vi "BotSpeak_AskDevice.vi"(3 "Bot Settings":T2={"Address"="", "Reply EOF"="", "Hardware"="", "Retries"=3, "Timeout"=10, "Open?"=FALSE}) -> (1 "Bot Settings out":T2)   [LabVIEW 2012]
uses:
  <userlib>/botspeak/VIs/Direct/BotSpeak_Control.ctl
  <vilib>/Platform/browser.llb/Open URL in Default Browser (string).vi
  <userlib>/botspeak/VIs/SubVIs/BotSpeak_Globals.vi
panel:
  out "Finished":bool
  in  "View":enum32{"Normal", "Testing"}(tab)
  out "Help":string
  in  "Hardware":u16(ring) items=["Arduino Uno", "BeagleBone Serial", "BeagleBone", "Console Only", "EV3", "EvalRIO", "Galileo", "Launchpad", "MyRIO", "PICAXE 80M", "Raspberry Pi", "Thymio"]
  in  "Done":bool
  in  "Cancel":bool
  in  "Connection":T1(tab)
  in  "IP Address":string(combo)
  in  "VISA":u16(ring)
  in  "Test":bool
  in  "Goto URL":bool
  out "URL":string
  out "Status":string
  out "firmware":string
  in  "Back":bool
  out "List":string[](array[string])
  # "For More Help:"
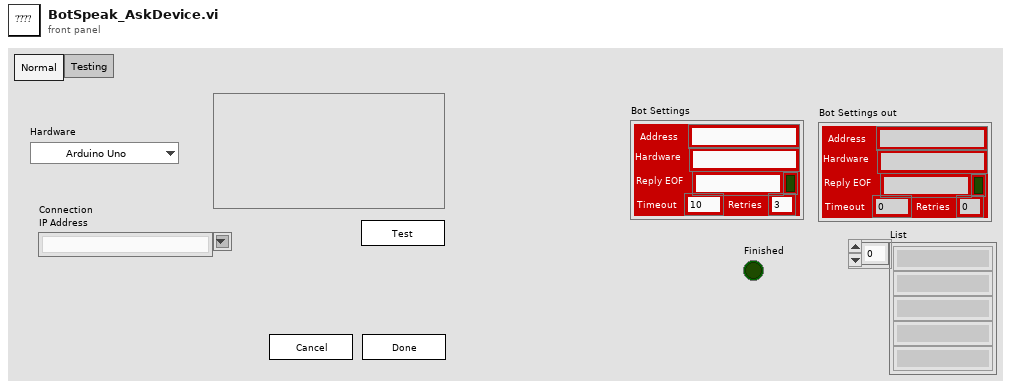
[diagram p1: front panel]
types:
  T1 = enum32{"TCPIP", "Serial", "Undefined", "Console"}
  T2 = typedef "BotSpeak_Control.ctl" = cluster{"Address":string, "Reply EOF":string, "Hardware":string, "Retries":i8, "Timeout":i32, "Open?":bool}
  T3 = typedef "BotSpeak.HardwareSpecs.ctl" = cluster{"Hardware Name":string, "Hardware URL":string, "ComType":enum16{"Undefined", "HTTP", "Serial", "TCPIP", "Console"}, "TCP Port":i32, "DefaultAddress":string, "Retries":i32, "Translate":enum16{"None", "Tiny", "URAPI"}, "MaxScriptSize":i32, "MaxVarNumber":i32, "StartupWait":i32, "Patience":i32, "Startup Patience":i32, "Hardware Help":string, "Com Protocol":string, "Translator":cluster{"BotSpeak CMD":string, "CMD out":string}[], "Init Code":string, "Variable Format":enum16{"INT", "FLOAT", "FIXED"}, "username":string, "password":string}
  T4 = enum16{"Undefined", "HTTP", "Serial", "TCPIP", "Console"}
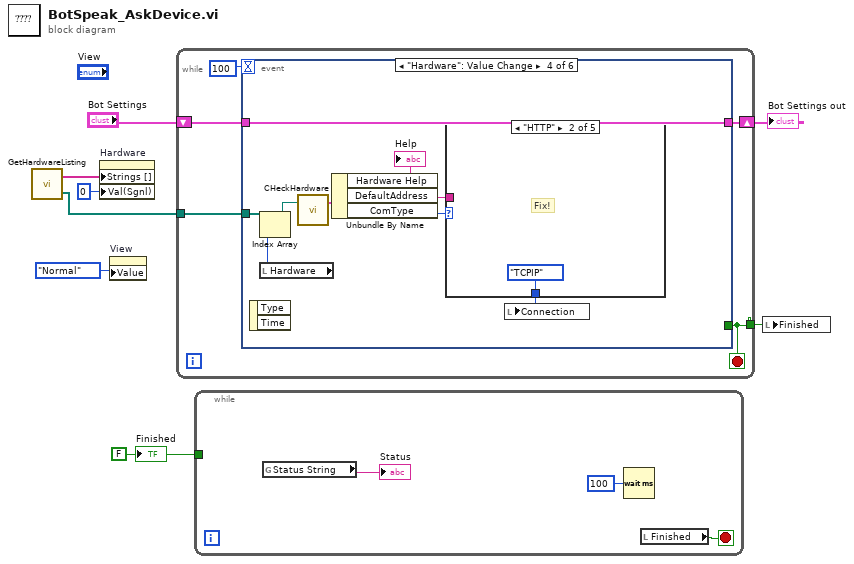
[diagram p0: block diagram]
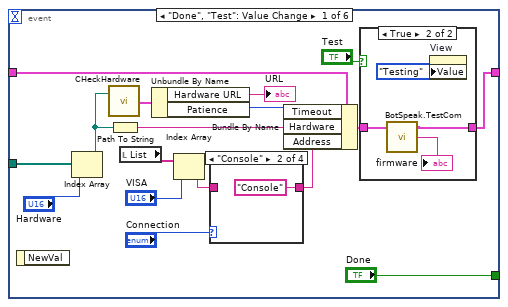
[diagram p2: hidden frame]
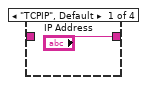
[diagram p3: hidden frame]
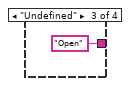
[diagram p4: hidden frame]
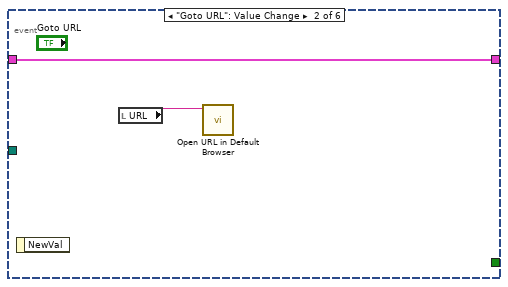
[diagram p7: hidden frame]
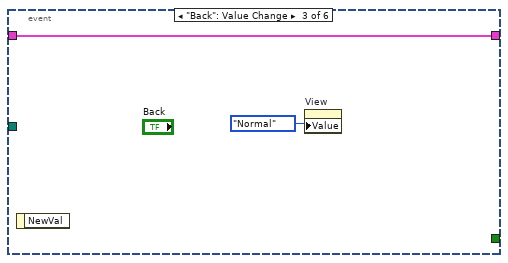
[diagram p8: hidden frame]
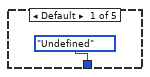
[diagram p9: hidden frame]
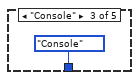
[diagram p10: hidden frame]
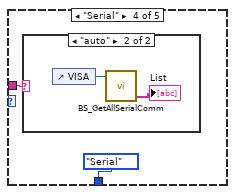
[diagram p11: hidden frame]
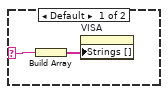
[diagram p12: hidden frame]
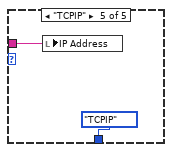
[diagram p13: hidden frame]
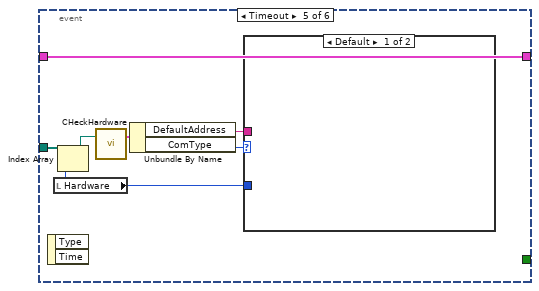
[diagram p14: hidden frame]
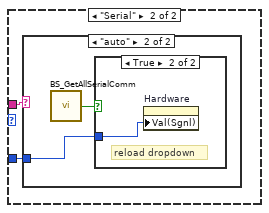
[diagram p15: hidden frame]
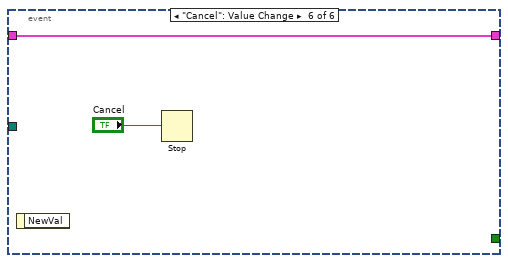
[diagram p18: hidden frame]
diagram:
  w3 = FALSE ("Finished")
  n1 = call <userlib>:"GetHardwareListing.vi"() -> ("Devices"=w1:path[], "Array"=w2:string[])  [unwired: 2 in]
  n2 = property on="Hardware" class="Ring (strict)"("Strings []"=w2, "Val(Sgnl)"=u16 0 ("Value (Signaling)")) -> ()  [unwired: 2 in, 2 out]
  n3 = property on="View" class="TabCtl (strict)"("Value"=enum32{"Normal", "Testing"}."Normal" ("View")) -> ()  [unwired: 2 in, 2 out]
  n4 = while {
    tunnel: w1 -> [w12]
    tunnel: [w9] -> w4
    shift-right: [w13] -> w8
    shift-left: "Bot Settings" -> [w11]
    stop <- w9 stop-if-true
    n5 = event shown="[3] \"Hardware\": Value Change" {
      selector: _ -> [_ _ _ _ _ _]
      dyn-events: _ -> [_ _ _ _ _ _]
      timeout: 100 -> [_ _ _ _ _ _]
      tunnel: w12 -> [w30 _ _ w52 w70 _]
      tunnel: w11 -> [w28 w40 w42 w44 w64 w76]
      tunnel: [w20 w40 w42 w44 w64 w76] -> w13
      tunnel: ["Done" _ _ _ _ _] -> w9
      event "Done", "Test": Value Change {
        n6 = event-data() -> ()  [unwired: 1 in, 1 out]
        n7 = Index Array(array=w30, index="Hardware") -> (element=w19:path)
        n8 = call <userlib>:"CHeckHardware.vi"("Hardware"=w19) -> ("HardwareSpecs"=w23:T3)  [unwired: 2 in]
        n9 = Path To String(path=w19) -> (string=w14:string)
        n10 = local read "List"() -> (w25:string[])
        n11 = Unbundle By Name(w23) -> ("Hardware URL"=→"URL":string, "Patience"=w15:i32)
        n12 = Index Array(array=w25, index="VISA") -> (element=w16:string)
        n13 = case shown="\"Console\"" "Connection" {
          tunnel: ["IP Address" "Console" ("Intf Inst Name") "Open" ("Intf Inst Name") w34] -> w17
          tunnel: w16 -> [_ _ _ w34]
          frame "TCPIP", Default {
          }
          frame "Console" {
          }
          frame "Undefined" {
          }
          frame "Serial" {
          }
        }
        n14 = Bundle By Name(cluster=w28, "Timeout"=w15, "Hardware"=w14, "Address"=w17) -> (w21:T2)
        n15 = case shown="True" "Test" {
          tunnel: w21 -> [w35 w38]
          tunnel: [w35 w37] -> w20
          frame False {
          }
          frame True {
            n16 = call <userlib>:"BotSpeak.TestCom.vi"("Bot Settings"=w38) -> ("Bot Settings out"=w37:T2, "firmware"=→"firmware":string)  [unwired: 1 in, 1 out]
            n17 = property on="View" class="TabCtl (strict)"("Value"=enum32{"Normal", "Testing"}."Testing" ("View")) -> ()  [unwired: 2 in, 2 out]
          }
        }
      }
      event "Goto URL": Value Change {
        n18 = event-data() -> ()  [unwired: 1 in, 1 out]
        n19 = local read "URL"() -> (w41:string)
        n20 = call-poly <vilib>:"Open URL in Default Browser.vi"("URL"=w41) -> ()  [unwired: 5 in, 2 out]
      }
      event "Back": Value Change {
        n21 = event-data() -> ()  [unwired: 1 in, 1 out]
        n22 = property on="View" class="TabCtl (strict)"("Value"=enum32{"Normal", "Testing"}."Normal" ("View")) -> ()  [unwired: 2 in, 2 out]
      }
      event "Hardware": Value Change {
        n23 = event-data() -> ()  [unwired: 1 in, 2 out]
        n24 = local read "Hardware"() -> (w46:u16)
        n25 = Index Array(array=w52, index=w46) -> (element=w51:path)
        n26 = call <userlib>:"CHeckHardware.vi"("Hardware"=w51) -> ("HardwareSpecs"=w50:T3)  [unwired: 2 in]
        n27 = Unbundle By Name(w50) -> ("Hardware Help"=→"Help":string, "DefaultAddress"=w47:string, "ComType"=w49:T4)
        n28 = case shown="\"HTTP\"" w49 {
          tunnel: [T1."Undefined" ("Connection") T1."TCPIP" ("Connection") T1."Console" ("Connection") enum32{"TCPIP", "Serial", "Undefined"}."Serial" ("Tabs") enum32{"TCPIP", "Serial", "Undefined"}."TCPIP" ("Tabs")] -> w48
          tunnel: w47 -> [_ _ _ w56 w62]
          frame Default {
          }
          frame "HTTP" {
            # "Fix!"
          }
          frame "Console" {
          }
          frame "Serial" {
            n29 = case shown="\"auto\"" w56 {
              selector: w56 -> [w59 _]
              frame Default {
                n30 = Build Array(w59) -> (w58:string[])
                n31 = property on="VISA" class="Ring (strict)"("Strings []"=w58) -> ()  [unwired: 2 in, 2 out]
              }
              frame "auto" {
                n32 = control-ref of="VISA"() -> (w61:refnum<vi>)
                n33 = call <userlib>:"BS_GetAllSerialComm.vi"("reference"=w61) -> ("List"=→"List":string[])  [unwired: 1 in, 2 out]
              }
            }
          }
          frame "TCPIP" {
            n34 = local write "IP Address"(w62) -> ()
          }
        }
        n35 = local write "Connection"(w48) -> ()
      }
      event Timeout {
        n36 = event-data() -> ()  [unwired: 1 in, 2 out]
        n37 = local read "Hardware"() -> (w65:u16)
        n38 = Index Array(array=w70, index=w65) -> (element=w69:path)
        n39 = call <userlib>:"CHeckHardware.vi"("Hardware"=w69) -> ("HardwareSpecs"=w68:T3)  [unwired: 2 in]
        n40 = Unbundle By Name(w68) -> ("DefaultAddress"=w66:string, "ComType"=w67:T4)
        n41 = case shown="Default" w67 {
          tunnel: w66 -> [_ w72]
          tunnel: w65 -> [_ w71]
          frame Default {
          }
          frame "Serial" {
            n42 = case shown="\"auto\"" w72 {
              tunnel: w71 -> [_ w73]
              frame Default {
              }
              frame "auto" {
                n43 = call <userlib>:"BS_GetAllSerialComm.vi"() -> ("new?"=w74:bool)  [unwired: 2 in, 2 out]
                n44 = case shown="True" w74 {
                  tunnel: w73 -> [_ w75]
                  frame False {
                  }
                  frame True {
                    # "reload dropdown"
                    n45 = property on="Hardware" class="Ring (strict)"("Val(Sgnl)"=w75) -> ()  [unwired: 2 in, 2 out]
                  }
                }
              }
            }
          }
        }
      }
      event "Cancel": Value Change {
        n46 = event-data() -> ()  [unwired: 1 in, 1 out]
        n47 = Stop(stop? (T)="Cancel") -> ()
      }
    }
  }
  "Bot Settings out" <- w8
  n48 = while {
    tunnel: w3 -> [_]
    stop <- w78 stop-if-true
    n49 = global read "BotSpeak_Globals.vi" "Status String"() -> (→"Status":string)
    n50 = Wait (ms)(milliseconds to wait=u32 100) -> ()  [unwired: 1 out]
    n51 = local read "Finished"() -> (w78:bool)
  }
  n52 = local write "Finished"(w4) -> ()
  "Finished" <- w3
